vi "CaseInsensitiveMatch.vi"(6 "error in":errorcluster, 9 "CaseStructure in":refnum<class "CaseStructure.lvclass">) -> (0 "error out":errorcluster, 3 "CaseStructure out":refnum<class "CaseStructure.lvclass">, 4 "Case Insensitive":bool)   [LabVIEW 2014, in "CaseStructure.lvclass"]
uses:
  CaseStructure.lvclass
  <vilib>/Utility/VariantDataType/VariantType.lvlib
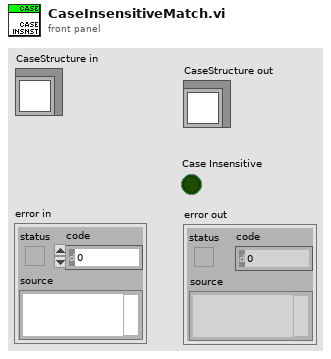
[diagram p1: front panel]
types:
  T1 = typedef "VariantType.lvlib/Type.ctl" = enum8{"Invalid Type", "Void", "I8", "I16", "I32", "I64", "U8", "U16", "U32", "U64", "Single Float", "Double Float", "Extended Float", "Single Complex", "Double Complex", "Extended Complex", "Enum U8", "Enum U16", "Enum U32", "Enum U64", "Single Float With Unit", "Double Float With Unit", "Extended Float With Unit", "Single Complex with Unit", "Double Complex with Unit", "Extended Complex with Unit", "Boolean", "String", "Path", "Picture", "Tag", "Array", "Cluster", "Variant", "LV Variant", "Waveform", "Timestamp", "Digital Waveform", "Digital Data", "ExpressData", "Refnum", "External Data", "VI", "Poly VI", "LabVIEW Class Instance", "Fixed Point"}
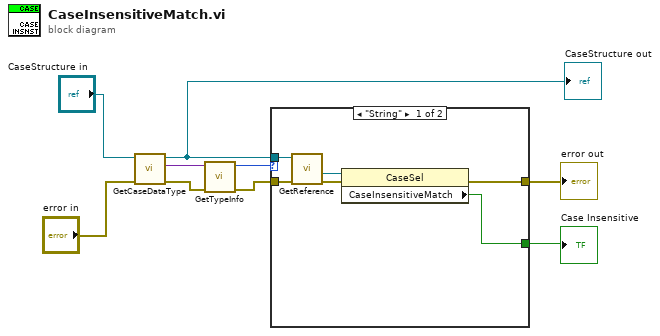
[diagram p0: block diagram]
diagram:
  n1 = call "GetCaseDataType.vi"("error in"="error in", "CaseStructure in"="CaseStructure in") -> ("error out"=w8:errorcluster, "Data Type"=w9:variant, "CaseStructure out"=w3:refnum<class "CaseStructure.lvclass">)  [unwired: 5 in]
  "CaseStructure out" <- w3
  n2 = call <vilib>:"GetTypeInfo.vi"("error in (no error)"=w8, "Variant"=w9) -> ("error out"=w6:errorcluster, "Type Enum"=w7:T1)  [unwired: 5 in, 3 out]
  n3 = case shown="\"String\"" w7 {
    tunnel: w6 -> [w14 w16]
    tunnel: [w11 w16] -> w2
    tunnel: w3 -> [w15 _]
    tunnel: [w10 _] -> w1
    frame "String" {
      n4 = call "GetReference.vi"("error in"=w14, "CaseStructure in"=w15) -> ("error out"=w12:errorcluster, "reference out"=w13:refnum<vi>)  [unwired: 7 in, 1 out]
      n5 = property class="CaseSel"(reference=w13, error in=w12) -> (error out=w11:errorcluster, "CaseInsensitiveMatch"=w10:bool)  [unwired: 1 out]
    }
    frame Default {
    }
  }
  "error out" <- w2
  "Case Insensitive" <- w1
